vi "Read_Joint_States.vi"(0 "error in":errorcluster, 2 "Units (deg)":enum16{"Radians", "Degrees"}(ring)=enum."Degrees", 3 "node":string) -> (1 "error out":errorcluster, 4 "Joint States":T1(array[cluster]))   [LabVIEW 2010]
doc: "Read all the current joint states (names, positions, velocity, and efforts)"
uses:
  ROS/Code/SubVIs/_ROSDirection.ctl
  ROS/Code/Console/Servers/ServerSubs/TopicDef.ctl
panel:
  out "Reply":string
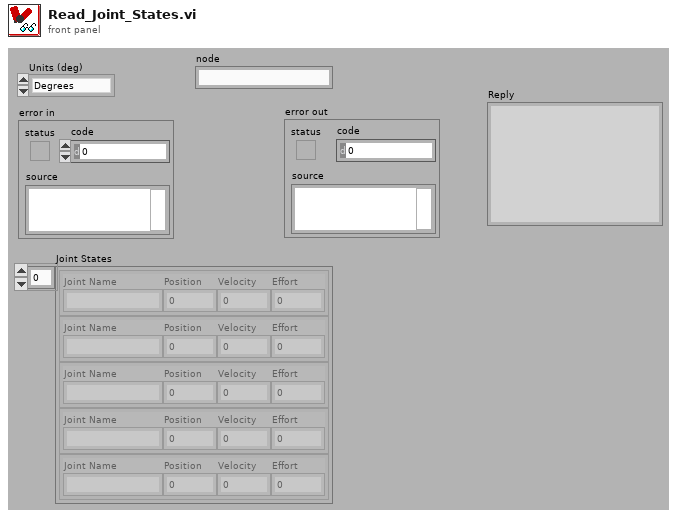
[diagram p1: front panel]
types:
  T1 = cluster{"Joint Name":string, "Position":dbl, "Velocity":dbl, "Effort":dbl}[]
  T2 = typedef "TopicDef.ctl" = cluster{"Topic":string, "Type":string, "Action":T3, "Update (ms)":u16, "write queue":u16}
  T3 = typedef "_ROSDirection.ctl" = enum16{"Node", "Publisher", "Subscriber", "Service Client"}
  T4 = typedef "_ROSControl.ctl" = cluster{"topic port":u16, "Node":string, "topic":string, "type":string, "node port":u32, "error ":errorcluster, "Direction":T3, "APIs":string[], "Update (ms)":u16, "write queue":u16}
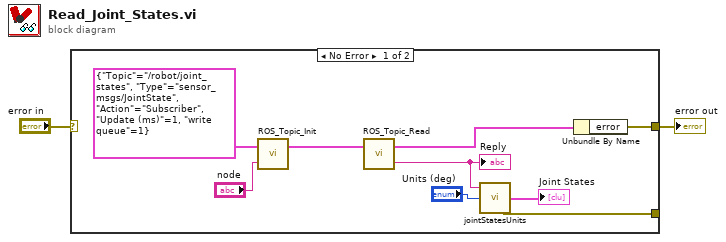
[diagram p0: block diagram]
diagram:
  n1 = case shown="No Error" "error in" {
    selector: "error in" -> [_ w12]
    tunnel: [w11 w12] -> w2
    tunnel: [w7 _] -> _
    frame No Error {
      n2 = call "ROS_Topic_Init.vi"("node"="node", "Definitions"=T2 {"Topic"="/robot/joint_states", "Type"="sensor_msgs/JointState", "Action"=enum."Subscriber", "Update (ms)"=1, "write queue"=1}) -> ("ROS out"=w9:T4)  [unwired: 1 in]
      n3 = call "ROS_Topic_Read.vi"("ROS in"=w9) -> ("Reply"=w4:string, "ROS out"=w8:T4)  [unwired: 1 in]
      "Reply" <- w4
      n4 = call "jointStatesUnits.vi"("Units (deg)"="Units (deg)", "msg in"=w4) -> ("error out"=w7:errorcluster, "Joint States"=→"Joint States":T1)  [unwired: 1 in, 1 out]
      n5 = Unbundle By Name(w8) -> ("error"=w11:errorcluster)
    }
    frame Error {
    }
  }
  "error out" <- w2
